vi "Configure Module.vi"(8 "error in (no error)":errorcluster, 10 "IOV ref in":refnum<k21>, 11 "Module Template in":refnum<class "9211.lvclass">) -> (0 "error out":errorcluster, 2 "IOV ref out":refnum<k21>, 3 "Module Template out":refnum<class "9211.lvclass">)   [LabVIEW 2017, in "Modules.lvlib" / "9211.lvclass"]
uses:
  9211.lvclass
  9211.lvclass/9211.ctl
  <resource>/objmgr/cRIO.rc
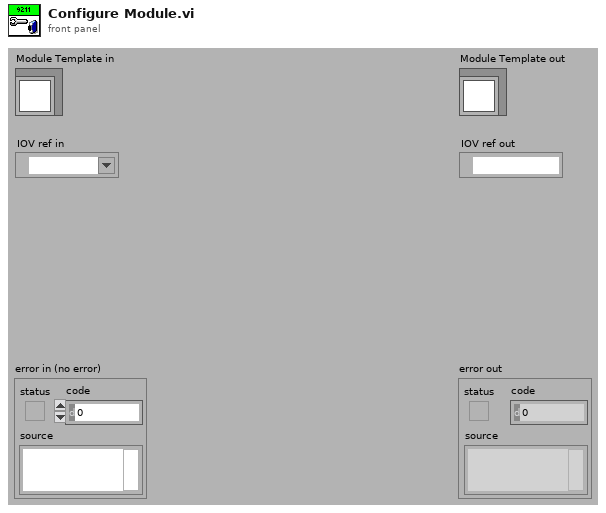
[diagram p1: front panel]
types:
  T1 = cluster{"Degree range":u32, "Thermocouple type":u32}[]
  T2 = cluster{"Degree range":u32, "Thermocouple type":u32}
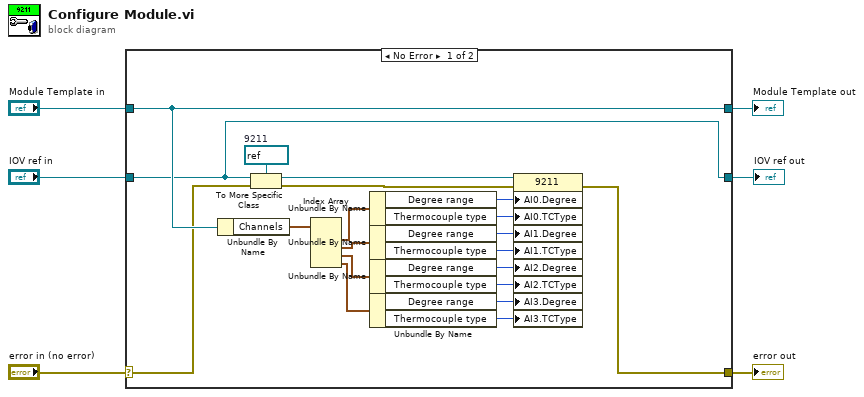
[diagram p0: block diagram]
diagram:
  n1 = case shown="No Error" "error in (no error)" {
    selector: "error in (no error)" -> [w25 w29]
    tunnel: [w21 w29] -> w5
    tunnel: [w26 w28] -> w3
    tunnel: "Module Template in" -> [w26 w28]
    tunnel: "IOV ref in" -> [w20 w27]
    tunnel: [w20 w27] -> w1
    frame No Error {
      w24 = refnum<k21> refnum  # 9211
      n2 = Unbundle By Name(w26) -> ("Channels"=w19:T1)
      n3 = To More Specific Class(target class=w24, reference=w20, error in=w25) -> (specific class reference=w23:refnum<k21>, error out=w22:errorcluster)
      n4 = Index Array(array=w19) -> (element #1=w18:T2, element #2=w9:T2, element #3=w8:T2, element #4=w7:T2)  [unwired: 4 in]
      n5 = Unbundle By Name(w18) -> ("Degree range"=w17:u32, "Thermocouple type"=w16:u32)
      n6 = Unbundle By Name(w9) -> ("Degree range"=w15:u32, "Thermocouple type"=w14:u32)
      n7 = Unbundle By Name(w8) -> ("Degree range"=w13:u32, "Thermocouple type"=w12:u32)
      n8 = Unbundle By Name(w7) -> ("Degree range"=w11:u32, "Thermocouple type"=w10:u32)
      n9 = property class="9211"(reference=w23, error in=w22, "AI0.Degree"=w17, "AI0.TCType"=w16, "AI1.Degree"=w15, "AI1.TCType"=w14, "AI2.Degree"=w13, "AI2.TCType"=w12, "AI3.Degree"=w11, "AI3.TCType"=w10) -> (error out=w21:errorcluster)  [unwired: 1 out]
    }
    frame Error {
    }
  }
  "error out" <- w5
  "Module Template out" <- w3
  "IOV ref out" <- w1
